vi "CreateActionMeasureState.vi"(7 "Enable":bool, 10 "Device":string, 11 "States in":string) -> (3 "States out":string)   [LabVIEW 2017, in "Measurement.Free.lvclass"]
uses:
  Measurement.Free.lvclass
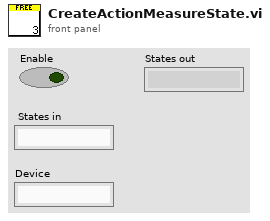
[diagram p1: front panel]
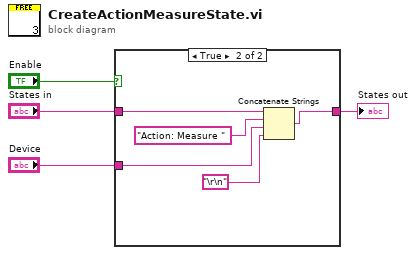
[diagram p0: block diagram]
diagram:
  n1 = case shown="True" "Enable" {
    tunnel: "States in" -> [w5 w10]
    tunnel: [w5 w8] -> w3
    tunnel: "Device" -> [_ w6]
    frame False {
    }
    frame True {
      n2 = Concatenate Strings(w10, "Action: Measure ", w6, "\r\n") -> (w8:string)
    }
  }
  "States out" <- w3
